vi "Read Pin.vi"(8 "error in (no error)":errorcluster, 9 "Pin 2":dbl caption="Pin", 10 "Port 4":dbl caption="Port", 11 "Simulado in":refnum<class "Simulado.lvclass">) -> (0 "error out":errorcluster, 3 "Simulado out":refnum<class "Simulado.lvclass">)   [LabVIEW 2020, in "Simulado.lvclass"]
uses:
  Simulado.lvclass
  Simulado.lvclass/Simulado.ctl
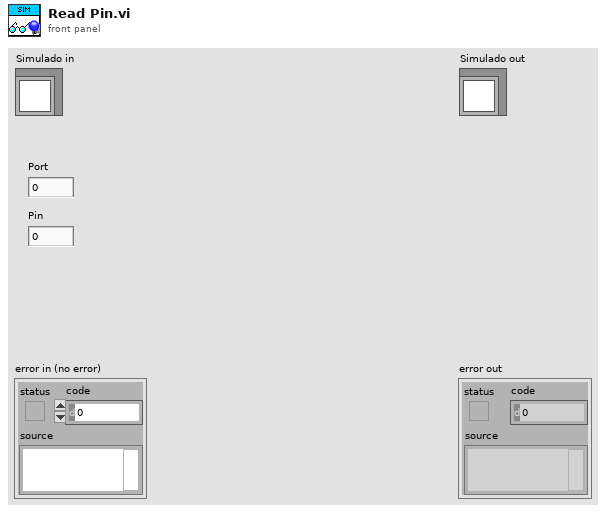
[diagram p1: front panel]
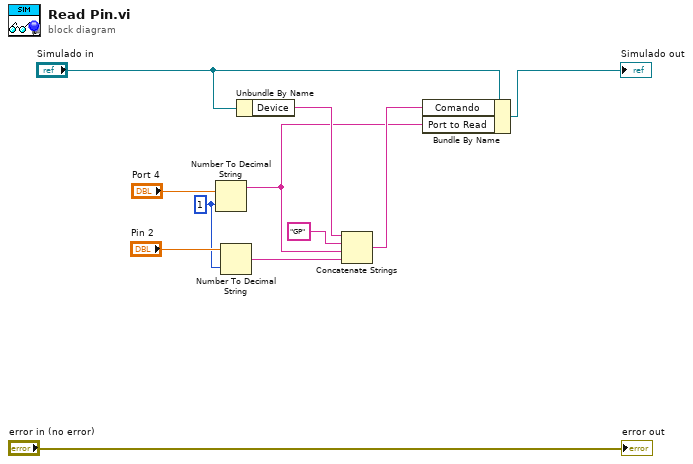
[diagram p0: block diagram]
diagram:
  w2 = i16 1 ("width (-)")
  n1 = Number To Decimal String(number="Port 4", width (-)=w2) -> (decimal integer string=w7:string)
  n2 = Number To Decimal String(number="Pin 2", width (-)=w2) -> (decimal integer string=w1:string)
  n3 = Unbundle By Name("Simulado in") -> ("Device"=w9:string)
  n4 = Concatenate Strings(w9, "GP" ("string"), w7, w1) -> (w8:string)
  n5 = Bundle By Name(cluster="Simulado in", "Comando"=w8, "Port to Read"=w7) -> (→"Simulado out":refnum<class "Simulado.lvclass">)
  "error out" <- "error in (no error)"
